vi "SpecAn Configure Common.vi"(0 "RFmx Handle In":refnum<k21>, 1 "Selector String":string, 5 "Common Configuration":T1={"Center Frequency (Hz)"=1000000000.0, "Reference Level (dBm)"=0.0, "External Attenuation (dB)"=0.0, "Enable Trigger?"=TRUE, "Digital Trigger Source"="PXI_Trig0", "Trigger Delay (s)"=0.0, "SelectedPorts"=""} {"Trigger Delay (s)" format="%.2p"; "External Attenuation (dB)" format="%.2f"; "Reference Level (dBm)" format="%.2f"; "Center Frequency (Hz)" format="%.6p"}, 11 "error in (no error)":errorcluster) -> (4 "RFmx Handle Out":refnum<k21>, 15 "error out":errorcluster)   [LabVIEW 2016, in "RFmxSpecAn.lvlib"]
uses:
  RFmxSpecAn.lvlib
  Common/SA Common Configuration.ctl
  <vilib>/RFmx/SpecAn/mx/RFmxSpecAn.llb/RFmxSpecAn Configure Digital Edge Trigger.vi
  <resource>/objmgr/RFmxSpecAn.rc
  Common/Common.lvlib
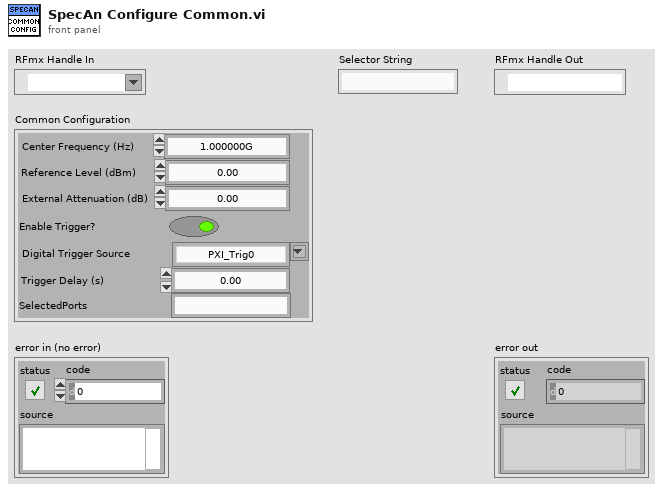
[diagram p1: front panel]
types:
  T1 = typedef "Common.lvlib/SA Common Configuration.ctl" = cluster{"Center Frequency (Hz)":dbl, "Reference Level (dBm)":dbl, "External Attenuation (dB)":dbl, "Enable Trigger?":bool, "Digital Trigger Source":string, "Trigger Delay (s)":dbl, "SelectedPorts":string}
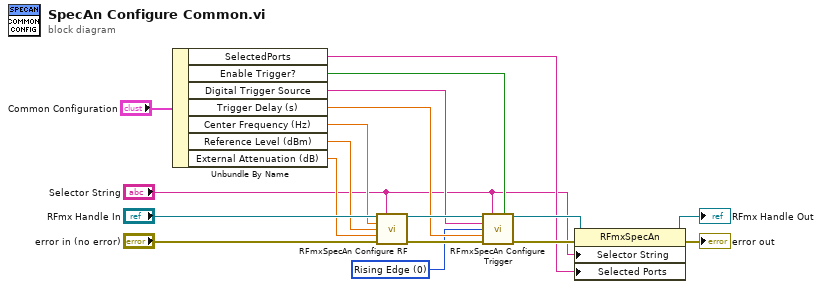
[diagram p0: block diagram]
diagram:
  w4 = 0 items=["Rising Edge", "Falling Edge"] ("Digital Edge")
  n1 = Unbundle By Name("Common Configuration") -> ("SelectedPorts"=w3:string, "Enable Trigger?"=w8:bool, "Digital Trigger Source"=w7:string, "Trigger Delay (s)"=w6:dbl, "Center Frequency (Hz)"=w14:dbl, "Reference Level (dBm)"=w13:dbl, "External Attenuation (dB)"=w12:dbl)
  n2 = call <vilib>:"RFmxSpecAn Configure RF.vi"("Instrument Handle In"="RFmx Handle In", "Selector String"="Selector String", "Center Frequency (Hz)"=w14, "Reference Level"=w13, "External Attenuation (dB)"=w12, "error in (no error)"="error in (no error)") -> ("Instrument Handle Out"=w18:refnum<k21>, "error out"=w17:errorcluster)  [unwired: 8 in]
  n3 = call-poly <vilib>:"RFmxSpecAn Configure Trigger.vi"("Instrument Handle In"=w18, "Selector String"="Selector String", "Enable Trigger?"=w8, "Digital Edge Source"=w7, "Digital Edge"=w4, "Trigger Delay (s)"=w6, "error in (no error)"=w17) -> ("Instrument Handle Out"=w5:refnum<k21>, "error out"=w10:errorcluster)  [unwired: 7 in]
  n4 = property class="RFmxSpecAn"(reference=w5, error in=w10, "Selector String"="Selector String", "Selected Ports"=w3) -> (reference out=→"RFmx Handle Out":refnum<k21>, error out=→"error out":errorcluster)
